vi "Automotive Dashboard Simulation (Arduino Nano & LabVIEW).VI"() -> ()   [LabVIEW 2020]
uses:
  <vilib>/Instr/_visa.llb/VISA Configure Serial Port (Instr).vi
panel:
  out "Over Heat !":bool
  out "Fuel level (Lit)":dbl(slide) scale=0.0..10.0
  out "°C":dbl
  out "Thermometer":dbl(slide) scale=0.0..100.0
  out "Time":string
  out "4":bool
  out "N":bool
  out "3":bool
  out "2":bool
  out "1":bool
  out "TAY SO":dbl
  out "COS":bool
  out "PHA":bool
  out "RIGHT":bool
  out "Vehical speed":i32(knob) scale=0.0..180.0
  out "Engine speed":i32(knob) scale=0.0..6000.0
  out "read buffer":string
  in  "VISA resource name":refnum<visa-resource-name>
  in  "stop":bool
  out "LEFT":bool
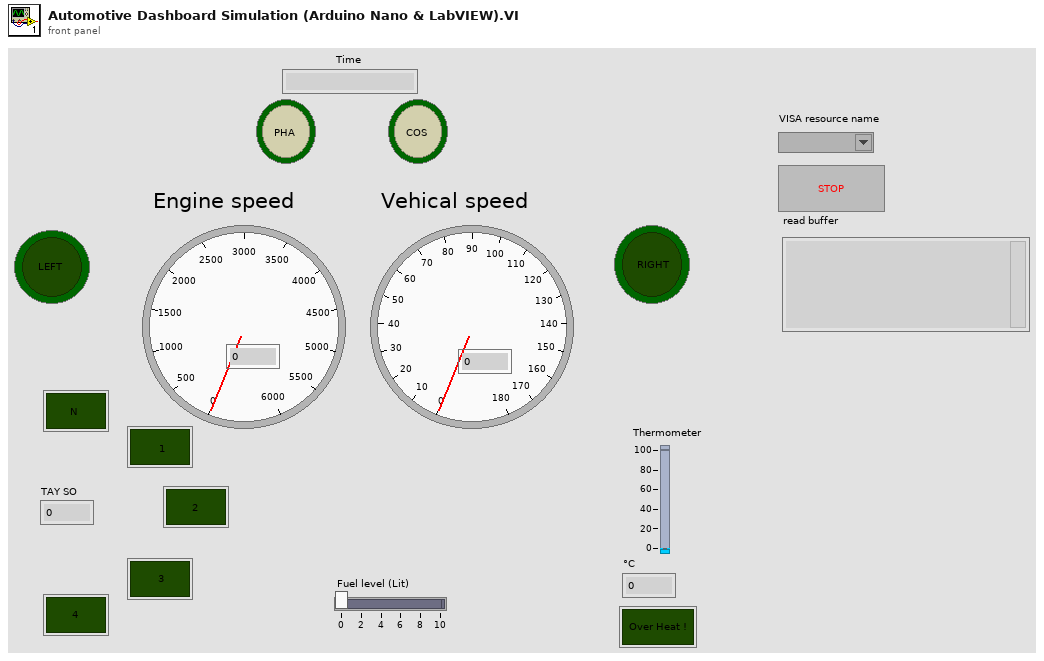
[diagram p1: front panel]
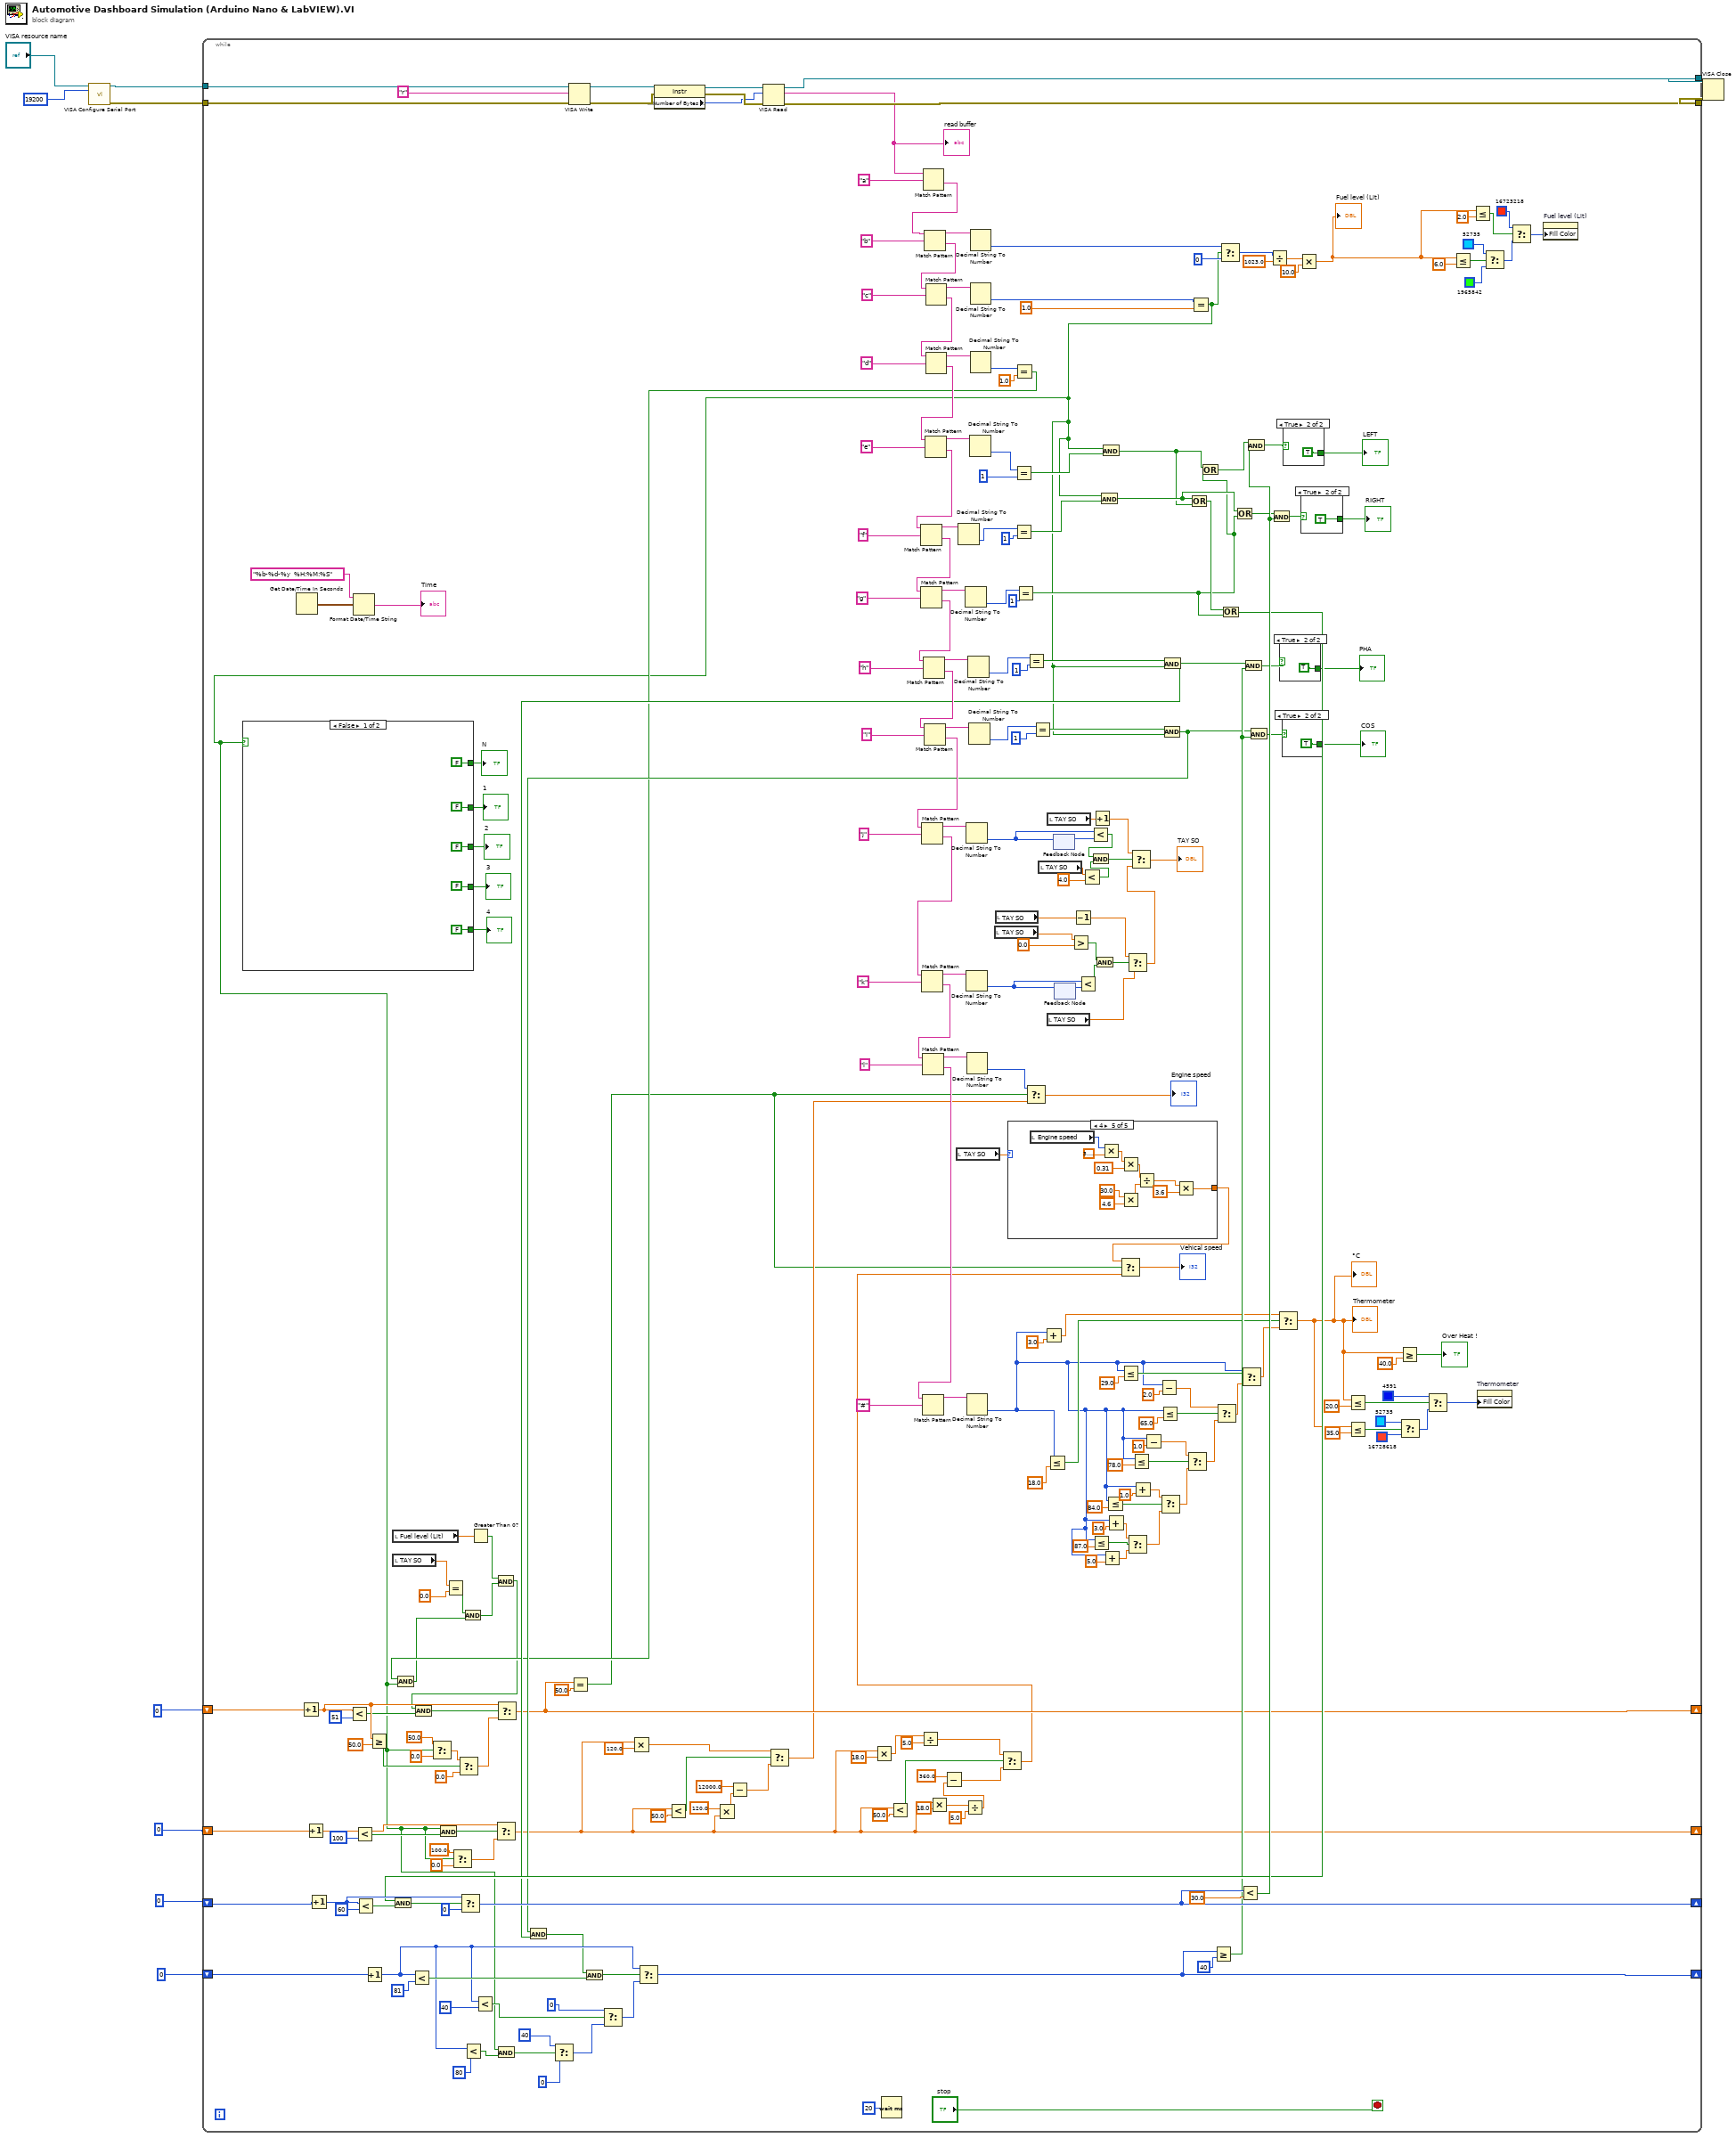
[diagram p0: block diagram]
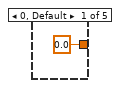
[diagram p2: hidden frame]
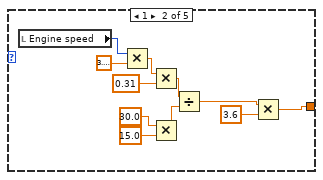
[diagram p3: hidden frame]
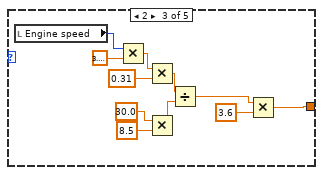
[diagram p4: hidden frame]
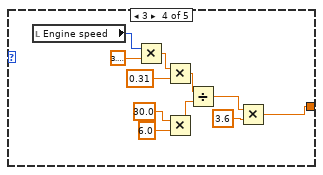
[diagram p5: hidden frame]
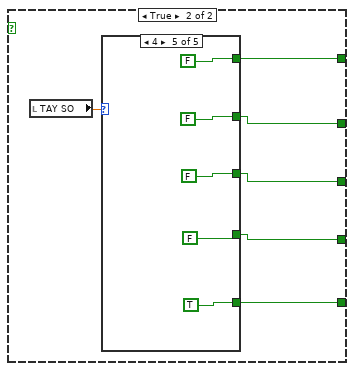
[diagram p6: hidden frame]
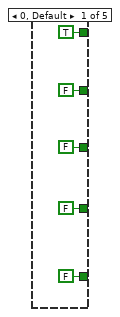
[diagram p7: hidden frame]
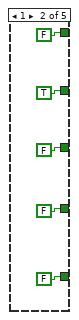
[diagram p8: hidden frame]
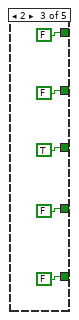
[diagram p9: hidden frame]
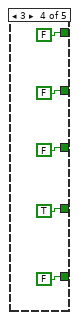
[diagram p10: hidden frame]
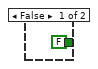
[diagram p11: hidden frame]
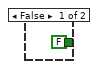
[diagram p12: hidden frame]
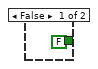
[diagram p13: hidden frame]
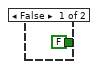
[diagram p14: hidden frame]
diagram:
  n1 = call-poly "VISA Configure Serial Port"("VISA resource name"="VISA resource name", "baud rate (9600)"=u32 19200) -> ("VISA resource name out"=w10:refnum<visa-resource-name>, "error out"=w8:errorcluster)  [unwired: 12 in]
  n2 = while {
    tunnel: w10 -> [w253]
    tunnel: [w269] -> w9
    tunnel: w8 -> [w252]
    tunnel: [w268] -> w7
    shift-right: [w239] -> _
    shift-left: 0 -> [w248]
    shift-right: [w186] -> _
    shift-left: 0 -> [w188]
    shift-right: [w60] -> _
    shift-left: 0 -> [w109]
    shift-right: [w88] -> _
    shift-left: 0 -> [w93]
    stop <- "stop" stop-if-true
    n3 = Get Date/Time In Seconds() -> (seconds since 1Jan1904=w162:timestamp)
    n4 = Increment(x=w93) -> (x+1=w80:dbl)
    n5 = Increment(x=w109) -> (x+1=w105:dbl)
    n6 = Increment(x=w248) -> (x+1=w242:i32)
    n7 = Less?(x=w80, y=51) -> (x < y?=w78:bool)
    n8 = Format Date/Time String(time format string (%c)="%b-%d-%y  %H:%M:%S", seconds (now)=w162) -> (date/time string=→"Time":string)  [unwired: 1 in]
    n9 = Less?(x=w105, y=100) -> (x < y?=w107:bool)
    n10 = Less?(x=w242, y=60) -> (x < y?=w244:bool)
    n11 = Increment(x=w188) -> (x+1=w192:i32)
    n12 = Greater Or Equal?(x=w80, y=50.0) -> (x >= y?=w79:bool)
    n13 = local read "Fuel level (Lit)"() -> (w47:dbl)
    n14 = local read "TAY SO"() -> (w72:dbl)
    n15 = Less?(x=w192, y=81) -> (x < y?=w199:bool)
    n16 = Equal?(x=w72, y=0.0 ("TAY SO")) -> (x = y?=w71:bool)
    n17 = Less?(x=w192, y=u8 80) -> (x < y?=w48:bool)
    n18 = Greater Than 0?(x=w47) -> (x > 0?=w46:bool)
    n19 = Less?(x=w192, y=u8 40) -> (x < y?=w196:bool)
    n20 = VISA Write(VISA resource name=w253, write buffer="r", error in (no error)=w252) -> (VISA resource name out=w251:refnum<visa-resource-name>, error out=w250:errorcluster)  [unwired: 1 out]
    n21 = property class="Instr"(reference=w251, error in=w250) -> (reference out=w267:refnum<visa-resource-name>, error out=w266:errorcluster, "Serial Settings:Number of Bytes at Serial Port"=w265:u32)
    n22 = VISA Read(VISA resource name=w267, byte count=w265, error in (no error)=w266) -> (VISA resource name out=w269:refnum<visa-resource-name>, read buffer=w259:string, error out=w268:errorcluster)  [unwired: 1 out]
    "read buffer" <- w259
    n23 = Wait (ms)(milliseconds to wait=u32 20) -> ()  [unwired: 1 out]
    n24 = Match Pattern(string=w259, regular expression="a") -> (after substring=w256:string)  [unwired: 1 in, 3 out]
    n25 = Match Pattern(string=w256, regular expression="b") -> (before substring=w261:string, after substring=w255:string)  [unwired: 1 in, 2 out]
    n26 = Match Pattern(string=w255, regular expression="c") -> (before substring=w260:string, after substring=w130:string)  [unwired: 1 in, 2 out]
    n27 = Match Pattern(string=w130, regular expression="d") -> (before substring=w132:string, after substring=w129:string)  [unwired: 1 in, 2 out]
    n28 = Match Pattern(string=w129, regular expression="e") -> (before substring=w258:string, after substring=w227:string)  [unwired: 1 in, 2 out]
    n29 = Match Pattern(string=w227, regular expression="f") -> (before substring=w236:string, after substring=w226:string)  [unwired: 1 in, 2 out]
    n30 = Match Pattern(string=w226, regular expression="g") -> (before substring=w235:string, after substring=w225:string)  [unwired: 1 in, 2 out]
    n31 = Match Pattern(string=w225, regular expression="h") -> (before substring=w232:string, after substring=w224:string)  [unwired: 1 in, 2 out]
    n32 = Match Pattern(string=w224, regular expression="i") -> (before substring=w231:string, after substring=w223:string)  [unwired: 1 in, 2 out]
    n33 = Match Pattern(string=w223, regular expression="j") -> (before substring=w228:string, after substring=w220:string)  [unwired: 1 in, 2 out]
    n34 = Match Pattern(string=w220, regular expression="k") -> (before substring=w222:string, after substring=w158:string)  [unwired: 1 in, 2 out]
    n35 = Match Pattern(string=w158, regular expression="l") -> (before substring=w159:string, after substring=w155:string)  [unwired: 1 in, 2 out]
    n36 = Match Pattern(string=w155, regular expression="#") -> (before substring=w157:string)  [unwired: 1 in, 3 out]
    n37 = local read "TAY SO"() -> (w53:dbl)
    n38 = Decimal String To Number(string=w236) -> (number=w216:i32)  [unwired: 2 in, 1 out]
    n39 = Decimal String To Number(string=w235) -> (number=w213:i32)  [unwired: 2 in, 1 out]
    n40 = Decimal String To Number(string=w228) -> (number=w183:i32)  [unwired: 2 in, 1 out]
    n41 = Decimal String To Number(string=w222) -> (number=w181:i32)  [unwired: 2 in, 1 out]
    n42 = Decimal String To Number(string=w159) -> (number=w87:i32)  [unwired: 2 in, 1 out]
    n43 = Decimal String To Number(string=w157) -> (number=w15:i32)  [unwired: 2 in, 1 out]
    n44 = Decimal String To Number(string=w232) -> (number=w204:i32)  [unwired: 2 in, 1 out]
    n45 = Decimal String To Number(string=w231) -> (number=w203:i32)  [unwired: 2 in, 1 out]
    n46 = Decimal String To Number(string=w258) -> (number=w246:i32)  [unwired: 2 in, 1 out]
    n47 = Decimal String To Number(string=w261) -> (number=w127:i32)  [unwired: 2 in, 1 out]
    n48 = Decimal String To Number(string=w260) -> (number=w124:i32)  [unwired: 2 in, 1 out]
    n49 = Decimal String To Number(string=w132) -> (number=w83:i32)  [unwired: 2 in, 1 out]
    n50 = local read "TAY SO"() -> (w168:dbl)
    n51 = local read "TAY SO"() -> (w178:dbl)
    n52 = case shown="4" w53 {
      tunnel: [0.0 w273 w284 w295 w306] -> w52
      frame 0, Default {
      }
      frame 1 {
        n53 = local read "Engine speed"() -> (w280:i32)
        n54 = Multiply(x=w280, y=3.141592653589793) -> (x*y=w281:dbl)
        n55 = Multiply(x=w281, y=0.31) -> (x*y=w283:dbl)
        n56 = Multiply(x=30.0, y=15.0) -> (x*y=w282:dbl)
        n57 = Divide(x=w283, y=w282) -> (x/y=w274:dbl)
        n58 = Multiply(x=w274, y=3.6) -> (x*y=w273:dbl)
      }
      frame 2 {
        n59 = local read "Engine speed"() -> (w291:i32)
        n60 = Multiply(x=w291, y=3.141592653589793) -> (x*y=w292:dbl)
        n61 = Multiply(x=w292, y=0.31) -> (x*y=w294:dbl)
        n62 = Multiply(x=30.0, y=8.5) -> (x*y=w293:dbl)
        n63 = Divide(x=w294, y=w293) -> (x/y=w285:dbl)
        n64 = Multiply(x=w285, y=3.6) -> (x*y=w284:dbl)
      }
      frame 3 {
        n65 = local read "Engine speed"() -> (w302:i32)
        n66 = Multiply(x=w302, y=3.141592653589793) -> (x*y=w303:dbl)
        n67 = Multiply(x=w303, y=0.31) -> (x*y=w305:dbl)
        n68 = Multiply(x=30.0, y=6.0) -> (x*y=w304:dbl)
        n69 = Divide(x=w305, y=w304) -> (x/y=w296:dbl)
        n70 = Multiply(x=w296, y=3.6) -> (x*y=w295:dbl)
      }
      frame 4 {
        n71 = local read "Engine speed"() -> (w313:i32)
        n72 = Multiply(x=w313, y=3.141592653589793) -> (x*y=w314:dbl)
        n73 = Multiply(x=w314, y=0.31) -> (x*y=w316:dbl)
        n74 = Multiply(x=30.0, y=4.6) -> (x*y=w315:dbl)
        n75 = Divide(x=w316, y=w315) -> (x/y=w307:dbl)
        n76 = Multiply(x=w307, y=3.6) -> (x*y=w306:dbl)
      }
    }
    n77 = Equal?(x=w246, y=1) -> (x = y?=w123:bool)
    n78 = Equal?(x=w216, y=1) -> (x = y?=w122:bool)
    n79 = Equal?(x=w83, y=1.0) -> (x = y?=w82:bool)
    n80 = Equal?(x=w213, y=1) -> (x = y?=w120:bool)
    n81 = Equal?(x=w204, y=1) -> (x = y?=w117:bool)
    n82 = Equal?(x=w203, y=1) -> (x = y?=w118:bool)
    n83 = local read "TAY SO"() -> (w172:dbl)
    n84 = Add(x=w15, y=3.0) -> (x+y=w40:dbl)
    n85 = local read "TAY SO"() -> (w176:dbl)
    n86 = Less Or Equal?(x=w15, y=18.0) -> (x <= y?=w42:bool)
    n87 = local read "TAY SO"() -> (w180:dbl)
    n88 = feedback #1() -> (w184:i32)  [unwired: 1 in]
    n89 = feedback-in #1(w183) -> ()
    n90 = feedback #2() -> (w182:i32)  [unwired: 1 in]
    n91 = feedback-in #2(w181) -> ()
    n92 = Greater?(x=w168, y=0.0) -> (0:w166:bool)
    n93 = Decrement(x=w178) -> (x-1=w177:dbl)
    n94 = Less?(x=w181, y=w182) -> (x < y?=w165:bool)
    n95 = Less?(x=w172, y=4.0) -> (x < y?=w174:bool)
    n96 = Less?(x=w183, y=w184) -> (x < y?=w171:bool)
    n97 = And(x=w171, y=w174) -> (x .and. y?=w170:bool)
    n98 = Less Or Equal?(x=w15, y=87.0) -> (x <= y?=w21:bool)
    n99 = Increment(x=w180) -> (x+1=w179:dbl)
    n100 = And(x=w166, y=w165) -> (x .and. y?=w164:bool)
    n101 = Add(x=w15, y=5.0) -> (x+y=w16:dbl)
    n102 = Less Or Equal?(x=w15, y=84.0) -> (x <= y?=w25:bool)
    n103 = Add(x=w15, y=3.0) -> (x+y=w18:dbl)
    n104 = Less Or Equal?(x=w15, y=29.0) -> (x <= y?=w37:bool)
    n105 = Select(t=w18, s=w21, f=w16) -> (s? t:f=w20:dbl)
    n106 = Select(t=w177, s=w164, f=w176) -> (s? t:f=w175:dbl)
    n107 = Select(t=w179, s=w170, f=w175) -> (s? t:f=→"TAY SO":dbl)
    n108 = Less Or Equal?(x=w15, y=78.0) -> (x <= y?=w31:bool)
    n109 = Add(x=w15, y=1.0) -> (x+y=w23:dbl)
    n110 = Subtract(x=w15, y=1.0) -> (x-y=w28:dbl)
    n111 = Subtract(x=w15, y=2.0) -> (x-y=w34:dbl)
    n112 = Less Or Equal?(x=w15, y=65.0) -> (x <= y?=w32:bool)
    n113 = Select(t=w23, s=w25, f=w20) -> (s? t:f=w14:dbl)
    n114 = Select(t=w28, s=w31, f=w14) -> (s? t:f=w27:dbl)
    n115 = Equal?(x=w124, y=1.0) -> (x = y?=w49:bool)
    n116 = case shown="False" w49 {
      tunnel: [FALSE ("N") w326] -> w114
      tunnel: [FALSE ("1") w325] -> w113
      tunnel: [FALSE ("2") w324] -> w112
      tunnel: [FALSE ("3") w323] -> w111
      tunnel: [FALSE ("4") w322] -> w110
      frame False {
      }
      frame True {
        n117 = local read "TAY SO"() -> (w327:dbl)
        n118 = case shown="4" w327 {
          tunnel: [TRUE ("N") FALSE ("N") FALSE ("N") FALSE ("N") FALSE ("N")] -> w326
          tunnel: [FALSE ("1") TRUE ("1") FALSE ("1") FALSE ("1") FALSE ("1")] -> w325
          tunnel: [FALSE ("2") FALSE ("2") TRUE ("2") FALSE ("2") FALSE ("2")] -> w324
          tunnel: [FALSE ("3") FALSE ("3") FALSE ("3") TRUE ("3") FALSE ("3")] -> w323
          tunnel: [FALSE ("4") FALSE ("4") FALSE ("4") FALSE ("4") TRUE ("4")] -> w322
          frame 0, Default {
          }
          frame 1 {
          }
          frame 2 {
          }
          frame 3 {
          }
          frame 4 {
          }
        }
      }
    }
    "N" <- w114
    "1" <- w113
    "2" <- w112
    "3" <- w111
    "4" <- w110
    n119 = And(x=w82, y=w49) -> (x .and. y?=w70:bool)
    n120 = Select(t=50.0, s=w49, f=0.0) -> (s? t:f=w74:dbl)
    n121 = And(x=w49, y=w107) -> (x .and. y?=w106:bool)
    n122 = Select(t=100.0, s=w49, f=0.0) -> (s? t:f=w94:dbl)
    n123 = Select(t=w74, s=w79, f=0.0) -> (s? t:f=w90:dbl)
    n124 = And(x=w71, y=w70) -> (x .and. y?=w45:bool)
    n125 = And(x=w46, y=w45) -> (x .and. y?=w44:bool)
    n126 = And(x=w44, y=w78) -> (x .and. y?=w77:bool)
    n127 = Select(t=w105, s=w106, f=w94) -> (s? t:f=w60:dbl)
    n128 = Select(t=w80, s=w77, f=w90) -> (s? t:f=w88:dbl)
    n129 = And(x=w49, y=w48) -> (x .and. y?=w50:bool)
    n130 = Select(t=u8 40, s=w50, f=u8 0) -> (s? t:f=w191:u8)
    n131 = Equal?(x=w88, y=50.0) -> (x = y?=w54:bool)
    n132 = Select(t=0, s=w196, f=w191) -> (s? t:f=w195:i32)
    n133 = Multiply(x=w60, y=120.0) -> (x*y=w101:dbl)
    n134 = Less?(x=w60, y=50.0) -> (x < y?=w103:bool)
    n135 = Multiply(x=120.0, y=w60) -> (x*y=w99:dbl)
    n136 = Subtract(x=12000.0, y=w99) -> (x-y=w97:dbl)
    n137 = Select(t=w101, s=w103, f=w97) -> (s? t:f=w85:dbl)
    n138 = Multiply(x=w60, y=18.0) -> (x*y=w65:dbl)
    n139 = Less?(x=w60, y=50.0) -> (x < y?=w67:bool)
    n140 = Divide(x=w65, y=5.0) -> (x/y=w64:dbl)
    n141 = Multiply(x=w60, y=18.0) -> (x*y=w58:dbl)
    n142 = Divide(x=w58, y=5.0) -> (x/y=w57:dbl)
    n143 = Subtract(x=360.0, y=w57) -> (x-y=w62:dbl)
    n144 = Select(t=w64, s=w67, f=w62) -> (s? t:f=w56:dbl)
    n145 = Select(t=w87, s=w54, f=w85) -> (s? t:f=→"Engine speed":dbl)
    n146 = And(x=w49, y=w122) -> (x .and. y?=w121:bool)
    n147 = And(x=w49, y=w123) -> (x .and. y?=w119:bool)
    n148 = Select(t=w52, s=w54, f=w56) -> (s? t:f=→"Vehical speed":dbl)
    n149 = And(x=w118, y=w49) -> (x .and. y?=w115:bool)
    n150 = And(x=w117, y=w49) -> (x .and. y?=w116:bool)
    n151 = And(x=w115, y=w116) -> (x .and. y?=w51:bool)
    n152 = And(x=w51, y=w199) -> (x .and. y?=w198:bool)
    n153 = Select(t=w192, s=w198, f=w195) -> (s? t:f=w186:i32)
    n154 = Or(x=w121, y=w119) -> (x .or. y?=w210:bool)
    n155 = Or(x=w119, y=w120) -> (x .or. y?=w212:bool)
    n156 = Greater Or Equal?(x=w186, y=u8 40) -> (x >= y?=w185:bool)
    n157 = Select(t=w34, s=w32, f=w27) -> (s? t:f=w36:dbl)
    n158 = Select(t=w127, s=w49, f=0) -> (s? t:f=w128:i32)
    n159 = Or(x=w210, y=w120) -> (x .or. y?=w209:bool)
    n160 = And(x=w209, y=w244) -> (x .and. y?=w243:bool)
    n161 = Select(t=w242, s=w243, f=0) -> (s? t:f=w239:i32)
    n162 = Or(x=w121, y=w120) -> (x .or. y?=w211:bool)
    n163 = Less?(x=w239, y=30.0) -> (x < y?=w215:bool)
    n164 = Select(t=w15, s=w37, f=w36) -> (s? t:f=w39:dbl)
    n165 = And(x=w116, y=w185) -> (x .and. y?=w202:bool)
    n166 = And(x=w212, y=w215) -> (x .and. y?=w238:bool)
    n167 = And(x=w115, y=w185) -> (x .and. y?=w201:bool)
    n168 = Divide(x=w128, y=1023.0) -> (x/y=w144:dbl)
    n169 = And(x=w211, y=w215) -> (x .and. y?=w219:bool)
    n170 = Select(t=w40, s=w42, f=w39) -> (s? t:f=w12:dbl)
    "Thermometer" <- w12
    "°C" <- w12
    n171 = case shown="True" w202 {
      tunnel: [FALSE ("Boolean") TRUE ("Boolean")] -> w206
      frame False {
      }
      frame True {
      }
    }
    "PHA" <- w206
    n172 = case shown="True" w201 {
      tunnel: [FALSE ("Boolean") TRUE ("Boolean")] -> w205
      frame False {
      }
      frame True {
      }
    }
    "COS" <- w205
    n173 = case shown="True" w238 {
      tunnel: [FALSE ("Boolean") TRUE ("Boolean")] -> w254
      frame False {
      }
      frame True {
      }
    }
    "LEFT" <- w254
    n174 = Multiply(x=w144, y=10.0) -> (x*y=w134:dbl)
    "Fuel level (Lit)" <- w134
    n175 = case shown="True" w219 {
      tunnel: [FALSE ("Boolean") TRUE ("Boolean")] -> w218
      frame False {
      }
      frame True {
      }
    }
    "RIGHT" <- w218
    n176 = Less Or Equal?(x=w12, y=20.0) -> (x <= y?=w153:bool)
    n177 = Less Or Equal?(x=w12, y=35.0) -> (x <= y?=w148:bool)
    n178 = Greater Or Equal?(x=w12, y=40.0) -> (x >= y?=→"Over Heat !":bool)
    n179 = Select(t=u32 52735 ("Fill Color"), s=w148, f=u32 16728618 ("Fill Color")) -> (s? t:f=w151:u32)
    n180 = Select(t=u32 4591 ("Fill Color"), s=w153, f=w151) -> (s? t:f=w150:u32)
    n181 = Less Or Equal?(x=w134, y=6.0) -> (x <= y?=w142:bool)
    n182 = Less Or Equal?(x=w134, y=2.0) -> (x <= y?=w140:bool)
    n183 = property on="Thermometer" class="Slide (strict)"("Fill Color"=w150) -> ()  [unwired: 2 in, 2 out]
    n184 = Select(t=u32 52735 ("Fill Color"), s=w142, f=u32 1965842 ("Fill Color")) -> (s? t:f=w141:u32)
    n185 = Select(t=u32 16723218 ("Fill Color"), s=w140, f=w141) -> (s? t:f=w133:u32)
    n186 = property on="Fuel level (Lit)" class="Slide (strict)"("Fill Color"=w133) -> ()  [unwired: 2 in, 2 out]
  }
  n187 = VISA Close(VISA resource name=w9, error in (no error)=w7) -> ()  [unwired: 1 out]
